vi "sv_Frequency Range to Band Number.vi"(1 "frequency range [Hz]":cluster{"low freq.":dbl, "high freq.":dbl}={"low freq."=1000.0, "high freq."=1000.0} {"high freq." min=0.001 format="%.2f"; "low freq." min=0.001 format="%.2f"}, 2 "bandwidth":T2(ring)=enum."1/3 octave", 3 "standard":T1) -> (0 "band number":cluster{"low band":i32, "high band":i32})   [LabVIEW 2017, in "SoundVib_Octave.lvlib"]
doc: "Converts the selected frequency range to the corresponding band number, based on the specified bandwidth and standard (ANSI or IEC).\nThe band number is based on the low and high bands specified in the frequency range cluster. A value of 0 corresponds to the reference frequency of the audio-frequency range, 1 kHz. Each successive value corresponds to the next fractional-octave band. Positive values cover the range above 1 kHz, and negative values cover the range below 1 kHz."
uses:
  <vilib>/addons/Sound and Vibration/svt_Octave/SoundVib_Octave.lvlib
  <vilib>/addons/_NISVFA/_Shared subVIs/Controls/svc_Octave Standard.ctl
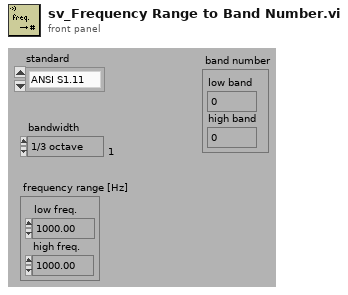
[diagram p1: front panel]
types:
  T1 = typedef "svc_Octave Standard.ctl" = enum16{"ANSI S1.11", "IEC 61260"}
  T2 = enum16{"1 octave", "1/3 octave", "1/6 octave", "1/12 octave", "1/24 octave", "1/48 octave", "1/96 octave"}
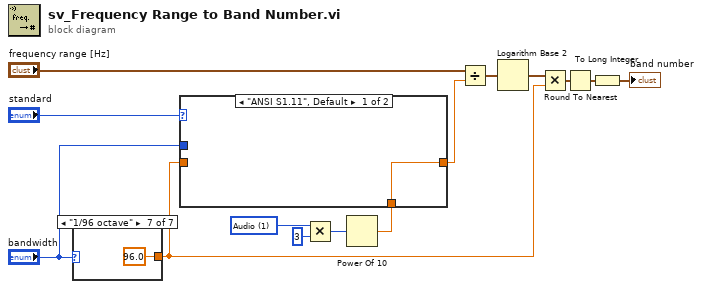
[diagram p0: block diagram]
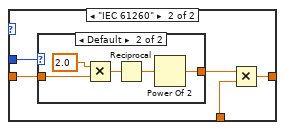
[diagram p2: hidden frame]
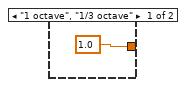
[diagram p3: hidden frame]
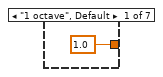
[diagram p4: hidden frame]
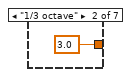
[diagram p5: hidden frame]
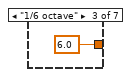
[diagram p6: hidden frame]
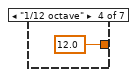
[diagram p7: hidden frame]
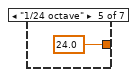
[diagram p8: hidden frame]
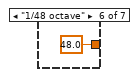
[diagram p9: hidden frame]
diagram:
  w8 = u16 1 items=["Infrasonic", "Audio", "Ultrasonic"] ("reference frequency range")
  n1 = case shown="\"1/96 octave\"" "bandwidth" {
    tunnel: [1.0 3.0 6.0 12.0 24.0 48.0 96.0] -> w1
    frame "1 octave", Default {
    }
    frame "1/3 octave" {
    }
    frame "1/6 octave" {
    }
    frame "1/12 octave" {
    }
    frame "1/24 octave" {
    }
    frame "1/48 octave" {
    }
    frame "1/96 octave" {
    }
  }
  n2 = Multiply(x=w8, y=u16 3) -> (x*y=w11:u16)
  n3 = Power Of 10(x=w11) -> (10^x=w9:dbl)
  n4 = case shown="\"ANSI S1.11\", Default" "standard" {
    tunnel: [w22 w26] -> w13
    tunnel: "bandwidth" -> [_ w27]
    tunnel: w1 -> [_ w24]
    tunnel: w9 -> [w22 w23]
    frame "ANSI S1.11", Default {
    }
    frame "IEC 61260" {
      n5 = case shown="Default" w27 {
        tunnel: [1.0 ("x") w33] -> w25
        tunnel: w24 -> [_ w30]
        frame "1 octave", "1/3 octave" {
        }
        frame Default {
          n6 = Multiply(x=2.0, y=w30) -> (x*y=w31:dbl)
          n7 = Reciprocal(x=w31) -> (1/x=w32:dbl)
          n8 = Power Of 2(x=w32) -> (2^x=w33:dbl)
        }
      }
      n9 = Multiply(x=w25, y=w23) -> (x*y=w26:dbl)
    }
  }
  n10 = Divide(x="frequency range [Hz]", y=w13) -> (x/y=w7:cluster{"low freq.":dbl, "high freq.":dbl})
  n11 = Logarithm Base 2(1:w7) -> (0:w6:cluster{"low freq.":dbl, "high freq.":dbl})
  n12 = Multiply(x=w6, y=w1) -> (x*y=w5:cluster{"low freq.":dbl, "high freq.":dbl})
  n13 = Round To Nearest(number=w5) -> (nearest integer value=w4:cluster{"low freq.":dbl, "high freq.":dbl})
  n14 = To Long Integer(number=w4) -> (32bit integer=→"band number":cluster{"low freq.":i32, "high freq.":i32})
